vi "Open.vi"(8 "error in (no error)":errorcluster, 11 "DeployTCPResource in":refnum<class "TCPResource.lvclass">) -> (0 "error out":errorcluster, 3 "DeployTCPResource out":refnum<class "TCPResource.lvclass">)   [LabVIEW 2020, in "PicoG-Core.lvlib" / "TCPResource.lvclass"]
uses:
  TCPResource.lvclass
  TCPResource.lvclass/TCPResource.ctl
  <vilib>/IlluminatedG/lv-stream-tcp/TCP Client/TCP Client.lvclass
  <vilib>/IlluminatedG/lv-stream/Endpoint/Endpoint.lvclass
  <vilib>/IlluminatedG/lv-stream-tcp/Stream-TCP.lvlib
  C:/Program Files (x86)/National Instruments/LabVIEW 2020/vi.lib/IlluminatedG/lv-stream/Connection/Connection.lvclass
  C:/Program Files (x86)/National Instruments/LabVIEW 2020/vi.lib/IlluminatedG/lv-stream/Endpoint/Endpoint.lvclass
  C:/Program Files (x86)/National Instruments/LabVIEW 2020/vi.lib/IlluminatedG/lv-stream-tcp/TCP Client/TCP Client.lvclass
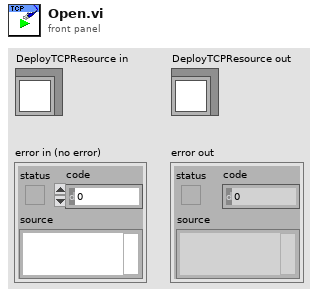
[diagram p1: front panel]
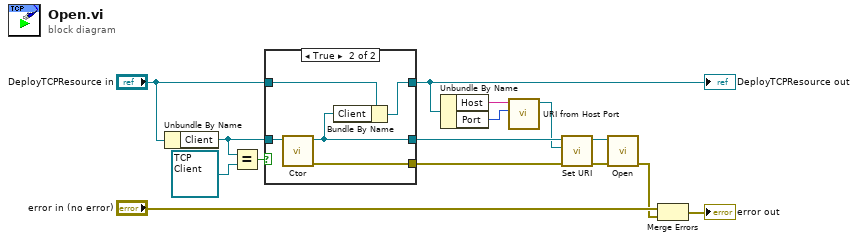
[diagram p0: block diagram]
diagram:
  n1 = Unbundle By Name("DeployTCPResource in") -> ("Client"=w13:refnum<class "TCP Client.lvclass">)
  n2 = Equal?(x=w13, y=refnum<class "TCP Client.lvclass"> refnum ("x")) -> (x = y?=w14:bool)
  n3 = case shown="True" w14 {
    tunnel: w13 -> [w16 w22]
    tunnel: "DeployTCPResource in" -> [w17 w21]
    tunnel: [w17 w20] -> w8
    tunnel: [w16 w19] -> w5
    tunnel: [_ w18] -> w4
    frame False {
    }
    frame True {
      n4 = call-dynamic "Ctor.vi"("TCP Client in"=w22) -> ("error out"=w18:errorcluster, "TCP Client out"=w19:refnum<class "TCP Client.lvclass">)  [unwired: 9 in]
      n5 = Bundle By Name(cluster=w21, "Client"=w19) -> (w20:refnum<class "TCPResource.lvclass">)
    }
  }
  "DeployTCPResource out" <- w8
  n6 = Unbundle By Name(w8) -> ("Host"=w7:string, "Port"=w6:u16)
  n7 = call <vilib>:"URI from Host Port.vi"("Port"=w6, "Host"=w7) -> ("URI"=w1:refnum<class "URI.lvclass">)  [unwired: 9 in]
  n8 = call <vilib>:"Set URI.vi"("error in (no error)"=w4, "URI"=w1, "Endpoint in"=w5) -> ("error out"=w3:errorcluster, "Endpoint out"=w2:refnum<class "TCP Client.lvclass">)  [unwired: 7 in]
  n9 = call <vilib>:"Open.vi"("error in (no error)"=w3, "Endpoint in"=w2) -> ("error out"=w10:errorcluster)  [unwired: 8 in, 1 out]
  n10 = Merge Errors("error in (no error)", w10) -> (→"error out":errorcluster)
